vi "Ritter Temperature Vapor Pressure Conversion.vi"(8 "error in (no error)":errorcluster, 11 "Temperature Value":dbl) -> (0 "error out":errorcluster, 3 "Water Vapor Pressure (in HG)":dbl)   [LabVIEW 2020]
uses:
  <vilib>/Analysis/NI_AALPro.lvlib
panel:
  out "Temperature Array":dbl[](array[numeric])
  out "Pressure Array":dbl[](array[numeric])
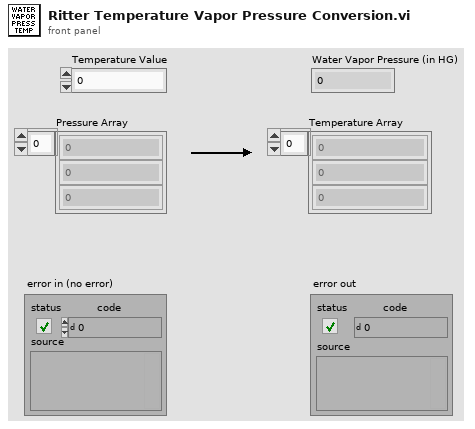
[diagram p1: front panel]
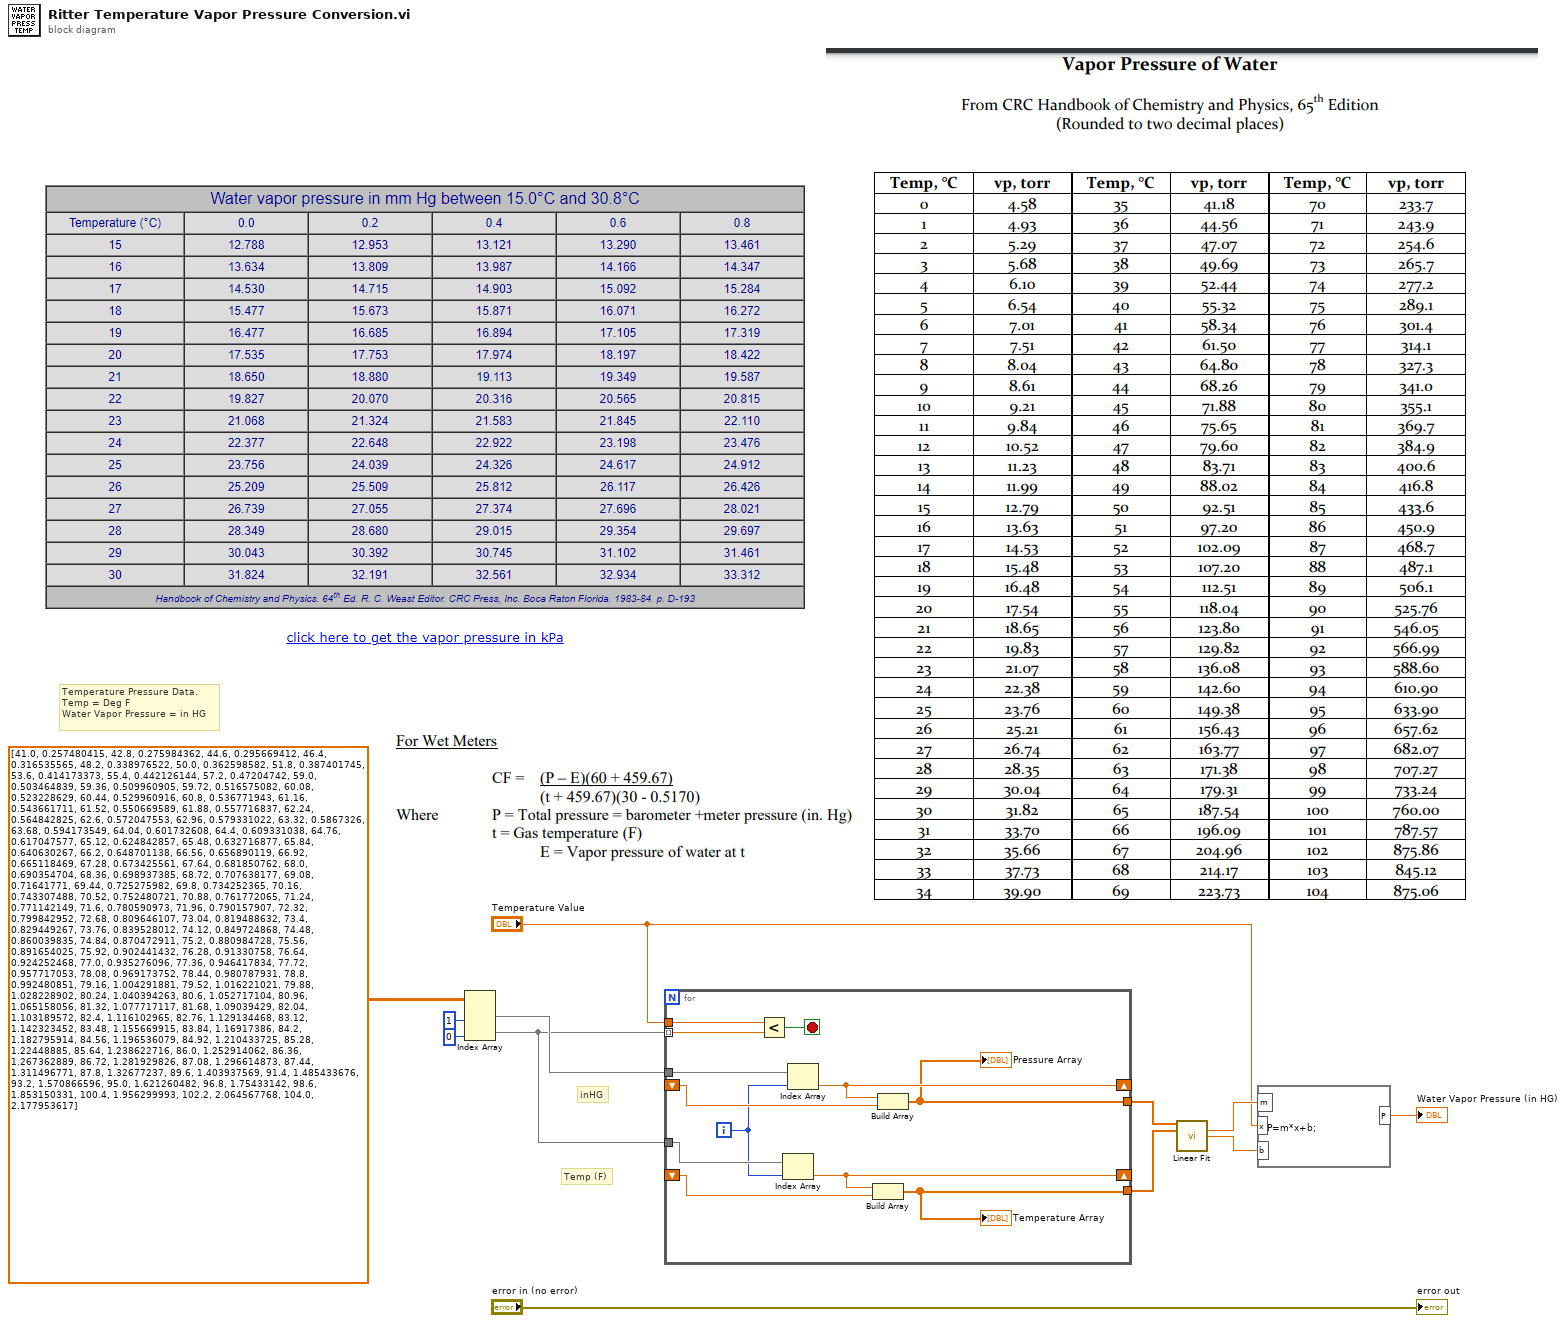
[diagram p0: block diagram]
diagram:
  # "Temp (F)"
  # "inHG"
  # "Temperature Pressure Data. \nTemp = Deg F\nWater Vapor Pressure = in HG"
  n1 = Index Array(array=dbl[][] [[41.0, 0.257480415], [42.8, 0.275984362], [44.6, 0.295669412], [46.4, 0.316535565], [48.2, 0.338976522], [50.0, 0.362598582], [51.8, 0.387401745], [53.6, 0.414173373], [55.4, 0.442126144], [57.2, 0.47204742], [59.0, 0.503464839], [59.36, 0.509960905], [59.72, 0.516575082], [60.08, 0.523228629], [60.44, 0.529960916], [60.8, 0.536771943], [61.16, 0.543661711], [61.52, 0.550669589], [61.88, 0.557716837], [62.24, 0.564842825], [62.6, 0.572047553], [62.96, 0.579331022], [63.32, 0.5867326], [63.68, 0.594173549], [64.04, 0.601732608], [64.4, 0.609331038], [64.76, 0.617047577], [65.12, 0.624842857], [65.48, 0.632716877], [65.84, 0.640630267], [66.2, 0.648701138], [66.56, 0.656890119], [66.92, 0.665118469], [67.28, 0.673425561], [67.64, 0.681850762], [68.0, 0.690354704], [68.36, 0.698937385], [68.72, 0.707638177], [69.08, 0.71641771], [69.44, 0.725275982], [69.8, 0.734252365], [70.16, 0.743307488], [70.52, 0.752480721], [70.88, 0.761772065], [71.24, 0.771142149], [71.6, 0.780590973], [71.96, 0.790157907], [72.32, 0.799842952], [72.68, 0.809646107], [73.04, 0.819488632], [73.4, 0.829449267], [73.76, 0.839528012], [74.12, 0.849724868], [74.48, 0.860039835], [74.84, 0.870472911], [75.2, 0.880984728], [75.56, 0.891654025], [75.92, 0.902441432], [76.28, 0.91330758], [76.64, 0.924252468], [77.0, 0.935276096], [77.36, 0.946417834], [77.72, 0.957717053], [78.08, 0.969173752], [78.44, 0.980787931], [78.8, 0.992480851], [79.16, 1.004291881], [79.52, 1.016221021], [79.88, 1.028228902], [80.24, 1.040394263], [80.6, 1.052717104], [80.96, 1.065158056], [81.32, 1.077717117], [81.68, 1.09039429], [82.04, 1.103189572], [82.4, 1.116102965], [82.76, 1.129134468], [83.12, 1.142323452], [83.48, 1.155669915], [83.84, 1.16917386], [84.2, 1.182795914], [84.56, 1.196536079], [84.92, 1.210433725], [85.28, 1.22448885], [85.64, 1.238622716], [86.0, 1.252914062], [86.36, 1.267362889], [86.72, 1.281929826], [87.08, 1.296614873], [87.44, 1.311496771], [87.8, 1.32677237], [89.6, 1.403937569], [91.4, 1.485433676], [93.2, 1.570866596], [95.0, 1.621260482], [96.8, 1.75433142], [98.6, 1.853150331], [100.4, 1.956299993], [102.2, 2.064567768], [104.0, 2.177953617]] ("all rows 2"), index (col) #1=1 ("disabled index (col)"), index (col) #2=0 ("index (col)")) -> (element #1=w10:dbl[], element #2=w1:dbl[])  [unwired: 2 in]
  n2 = for {
    tunnel: w1 -> [w23] mode=indexing
    tunnel: "Temperature Value" -> [w15]
    tunnel: w10 -> [w22]
    shift-right: [w21] -> _
    shift-left: _ -> [w20]
    tunnel: w1 -> [w19]
    shift-right: [w17] -> _
    shift-left: _ -> [w16]
    tunnel: [w14] -> w5
    tunnel: [w13] -> w6
    i -> [w18]
    stop <- w24 stop-if-true
    n3 = Less?(x=w15, y=w23) -> (x < y?=w24:bool)
    n4 = Index Array(array=w19, index=w18) -> (element=w17:dbl)
    n5 = Index Array(array=w22, index=w18) -> (element=w21:dbl)
    n6 = Build Array(w17, w16) -> (w13:dbl[])
    "Temperature Array" <- w13
    n7 = Build Array(w21, w20) -> (w14:dbl[])
    "Pressure Array" <- w14
  }
  n8 = call <vilib>:"Linear Fit.vi"("Y"=w5, "X"=w6) -> ("slope"=w8:dbl, "intercept"=w9:dbl)  [unwired: 9 in, 3 out]
  n9 = formula code="P=m*x+b;"("m"=w8, "b"=w9, "x"="Temperature Value") -> ("P"=→"Water Vapor Pressure (in HG)":dbl)
  "error out" <- "error in (no error)"
